vi "Denoise - Image.vi"() -> ()   [LabVIEW 2023]
doc: "This example shows how to reduce noise of an image with the WA Denoise VI. The flower image is contaminated by some Gaussian white noise with a standard deviation 5. This example uses the undecimated wavelet transform-based method to denoise the image.\n\n<b>Instructions:</b>\n1) Run this VI.\n2) Compare the noisy image and denoised image with different settings."
uses:
  <vilib>/addons/Wavelet Analysis/typedefs.llb/WA Data.ctl
  <vilib>/addons/Wavelet Analysis/application.llb/WA Denoise (UWT 2D Array).vi
  <vilib>/addons/_Advanced Signal Processing/NI_AdvSigProcWA.lvlib
  <vilib>/Analysis/NI_AALBase.lvlib
panel:
  in  "Threshold settings":T1={"Thresholding Rule"=enum."SURE", "Rescaling Method"=enum."Single level", "Soft Threshold?"=TRUE}
  out "Denoised Image":dbl[][](graph)
  out "Noisy Image":dbl[][](graph)
  in  "Wavelet":u16(ring) items=["db02"=0, "db03"=1, "db04"=2, "db05"=3, "db06"=4, "db07"=5, "db08"=6, "db09"=7, "db10"=8, "db11"=9, "db12"=10, "db13"=11, "db14"=12, "Haar"=13, "bior1_3"=14, "bior1_5"=15, "bior2_2"=16, "bior2_4"=17, "bior2_6"=18, "bior2_8"=19, "bior3_1"=20, "bior3_3"=21, "bior3_5"=22, "bior3_7"=23, "bior3_9"=24, "bior4_4 (FBI)"=25, "bior5_5"=38, "bior6_8"=39, "coif1"=26, "coif2"=27, "coif3"=28, "coif4"=29, "coif5"=30, "sym2"=31, "sym3"=32, "sym4"=33, "sym5"=34, "sym6"=35, "sym7"=36, "sym8"=37]
  in  "Levels":i32=4
  # "Overview: Shows how to reduce noise of an image with the WA Denoise VI. The flower image is contaminated by some Gaussian white noise with a standard deviation 5. This example uses the undecimated wavelet transform-based method to denoise the image.\nRequirements: LabVIEW Full Development System, Advanced Signal Processing Toolkit\nInstructions: \n1. Run this VI.\n2. Compare the noisy image and denoised image with different settings."
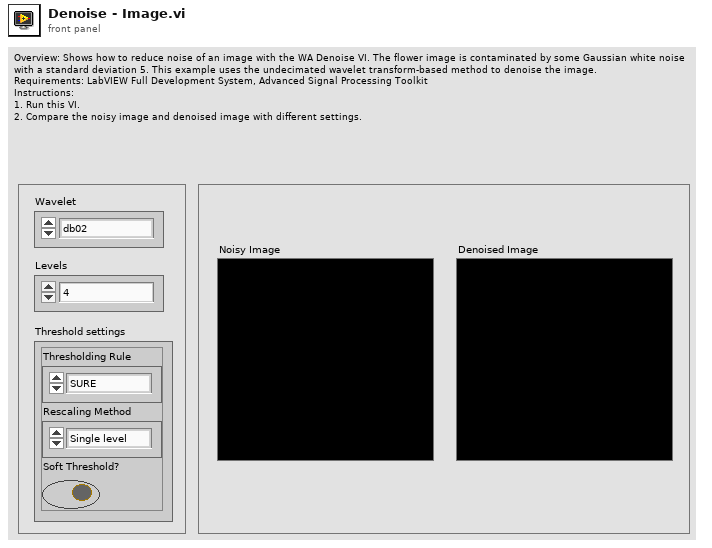
[diagram p1: front panel]
types:
  T1 = cluster{"Thresholding Rule":enum16{"SURE", "Hybrid", "Universal", "Minimax"}, "Rescaling Method":enum16{"One", "Single level", "Multiple levels"}, "Soft Threshold?":bool}
  T2 = typedef "NI_AdvSigProcWA.lvlib/WA Data.ctl" = u16
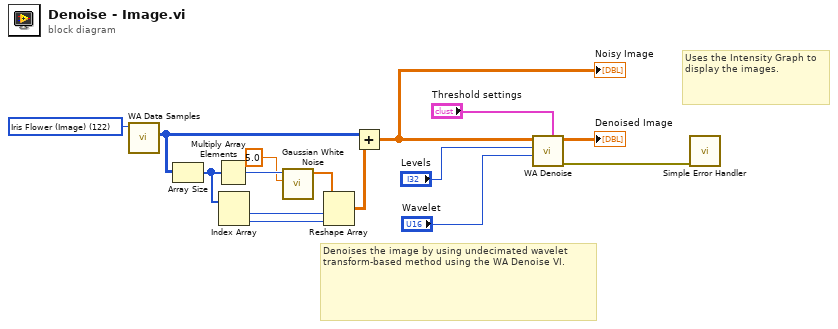
[diagram p0: block diagram]
diagram:
  w2 = T2 122 items=["1D Example Data"=100, "-"=101, "Doppler"=102, "HOP"=103, "TF Sine"=104, "Noisy Doppler"=105, "Sea Temperature"=106, "Sp500"=107, "Power Line"=108, "Engine Knocking"=109, "HeaviSine"=110, "Bumps"=111, "Blocks"=112, "Piece Regular"=113, "HypChirps"=114, "LinChirps"=115, "Chirps"=116, "Piece Polynomial"=117, "ECG"=131, "-"=118, "2D Example Data"=119, "-"=120, "Finger Print (Image)"=121, "Iris Flower (Image)"=122, "Mammogram (Image)"=123, "Lake (Image)"=127, "Two Can 1 (Image)"=132, "Two Can 2 (Image)"=133, "Camera Man (Image)"=134] ("data")
  # "Uses the Intensity Graph to display the images."
  # "Denoises the image by using undecimated wavelet transform-based method using the WA Denoise VI."
  n1 = call <vilib>:"WA Data Samples.vi"("data"=w2) -> ("image"=w8:u8[][])  [unwired: 10 out]
  n2 = Array Size(array=w8) -> (size(s)=w14:i32[])
  n3 = Multiply Array Elements(1:w14) -> (0:w15:i32)
  n4 = Index Array(array=w14) -> (element #1=w13:i32, element #2=w12:i32)  [unwired: 2 in]
  n5 = call <vilib>:"Gaussian White Noise.vi"("standard deviation"=5.0, "samples"=w15) -> ("Gaussian noise pattern"=w3:dbl[])  [unwired: 8 in, 1 out]
  n6 = Reshape Array(w3, w13, w12) -> (w11:dbl[][])
  n7 = Add(x=w8, y=w11) -> (x+y=w5:dbl[][])
  "Noisy Image" <- w5
  n8 = call-poly <vilib>:"WA Denoise.vi"("threshold settings"="Threshold settings", "wavelet"="Wavelet", "levels"="Levels", "signal"=w5) -> ("error out"=w1:errorcluster, "denoised signal"=→"Denoised Image":dbl[][])  [unwired: 1 in, 5 out]
  n9 = call <vilib>:"Simple Error Handler.vi"("error in (no error)"=w1) -> ()  [unwired: 4 in, 5 out]
